vi "Configure System Tray.vi"(8 "error in (no error)":errorcluster, 11 "Assert Startup UI in":refnum<class "Assert Startup UI.lvclass">) -> (0 "error out":errorcluster, 3 "Assert Startup UI out":refnum<class "Assert Startup UI.lvclass">, 5 "Notify Icon Event":refnum<user-event>)   [LabVIEW 2016, in "Assert API Components.lvlib" / "Assert Startup UI.lvlib" / "Assert Startup UI.lvclass"]
doc: "Sets up a system tray event and configures the icon and menu"
uses:
  Assert Startup UI.lvclass
  System Tray/Public/Controls/Notify Event.ctl
  System Tray/Public/Controls/Notify Event Type.ctl
  Assert Startup UI.lvclass/Assert Startup UI.ctl
  System Tray/Public/Tray Icon/Set Tray Notification Icon Poly/Set Tray Icon (file).vi
  System Tray/NotifyIcon.lvclass
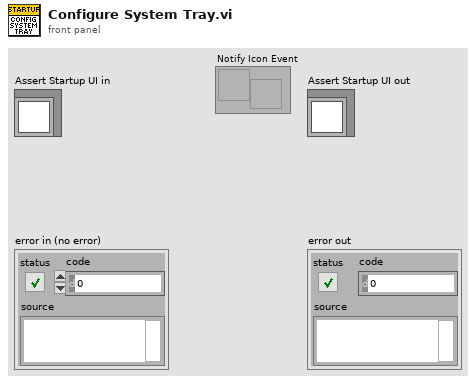
[diagram p1: front panel]
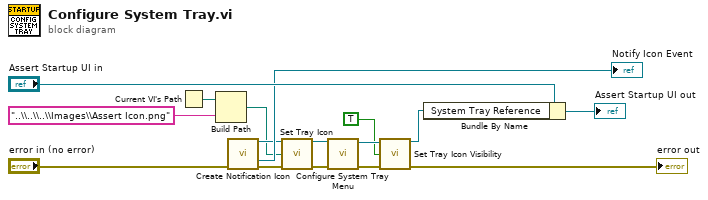
[diagram p0: block diagram]
diagram:
  n1 = Current VI's Path() -> (path=w4:path)
  n2 = Build Path(base path=w4, name or relative path="..\\..\\..\\Images\\Assert Icon.png") -> (appended path=w2:path)
  n3 = call "Create Notification Icon.vi"("error in (no error)"="error in (no error)") -> ("NotifyIcon out"=w12:refnum<class "NotifyIcon.lvclass">, "Notify Icon Event"=→"Notify Icon Event":refnum<user-event>, "error out"=w11:errorcluster)  [unwired: 12 out]
  n4 = call-poly "Set Tray Icon.vi"("NotifyIcon in"=w12, "Image file"=w2, "error in (no error)"=w11) -> ("NotifyIcon out"=w10:refnum<class "NotifyIcon.lvclass">, "error out"=w9:errorcluster)  [unwired: 11 out]
  n5 = call "Configure System Tray Menu.vi"("error in (no error)"=w9, "NotifyIcon in"=w10) -> ("error out"=w7:errorcluster, "NotifyIcon out"=w8:refnum<class "NotifyIcon.lvclass">)  [unwired: 8 in]
  n6 = call "Set Tray Icon Visibility.vi"("NotifyIcon in"=w8, "Show Tray Icon"=TRUE, "error in (no error)"=w7) -> ("NotifyIcon out"=w5:refnum<class "NotifyIcon.lvclass">, "error out"=→"error out":errorcluster)  [unwired: 11 out]
  n7 = Bundle By Name(cluster="Assert Startup UI in", "System Tray Reference"=w5) -> (→"Assert Startup UI out":refnum<class "Assert Startup UI.lvclass">)
